vi "Reserve Registered Sessions.vi"(6 "timeout (ms)":i32, 8 "error in (no error)":errorcluster, 9 "instrument type id":string) -> (0 "error out":errorcluster, 3 "session reservation out":refnum<class "Session Reservation.lvclass">)   [LabVIEW 2020, in "MeasurementLink Session Management.lvlib" / "Session Reservation.lvclass"]
doc: "Reserves all registered session(s) with the specified <b>instrument type id</b>. If the <b>instrument type id</b> is an empty string, reserves all registered sessions for all instrument types."
uses:
  Session Reservation.lvclass
  MeasurementLink Session Management Client/RPC Messages/ni_measurementlink_sessionmanagement_v1_ReserveAllRegisteredSessionsRequest.ctl
  MeasurementLink Session Management Client/RPC Messages/ni_measurementlink_PinMapContext.ctl
  IReservationObserver/IReservationObserver.lvclass
  Session Reservation.lvclass/Session Reservation.ctl
  MeasurementLink Session Management Client/MeasurementLink Session Management Client.lvlib
  MeasurementLink Session Management Client Wrapper/MeasurementLink Session Management Client Wrapper.lvlib
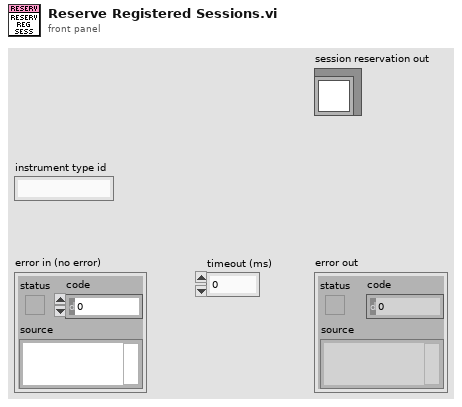
[diagram p1: front panel]
types:
  T1 = typedef "MeasurementLink Session Management Client.lvlib/ni_measurementlink_PinMapContext.ctl" = cluster{"pin_map_id":string, "sites":i32[]}
  T2 = typedef "MeasurementLink Session Management Client.lvlib/ni_measurementlink_sessionmanagement_v1_ReserveAllRegisteredSessionsRequest.ctl" = cluster{"timeout_in_milliseconds":i32, "instrument_type_id":string}
  T3 = typedef "MeasurementLink Session Management Client.lvlib/ni_measurementlink_sessionmanagement_v1_ReserveAllRegisteredSessionsResponse.ctl" = cluster{"sessions":T4[]}
  T4 = typedef "MeasurementLink Session Management Client.lvlib/ni_measurementlink_sessionmanagement_v1_SessionInformation.ctl" = cluster{"session":T5, "resource_name":string, "channel_list":string, "instrument_type_id":string, "session_exists":bool, "channel_mappings":T6[]}
  T5 = typedef "MeasurementLink Session Management Client.lvlib/nidevice_grpc_Session.ctl" = cluster{"name":string}
  T6 = typedef "MeasurementLink Session Management Client.lvlib/ni_measurementlink_sessionmanagement_v1_ChannelMapping.ctl" = cluster{"pin_or_relay_name":string, "site":i32, "channel":string}
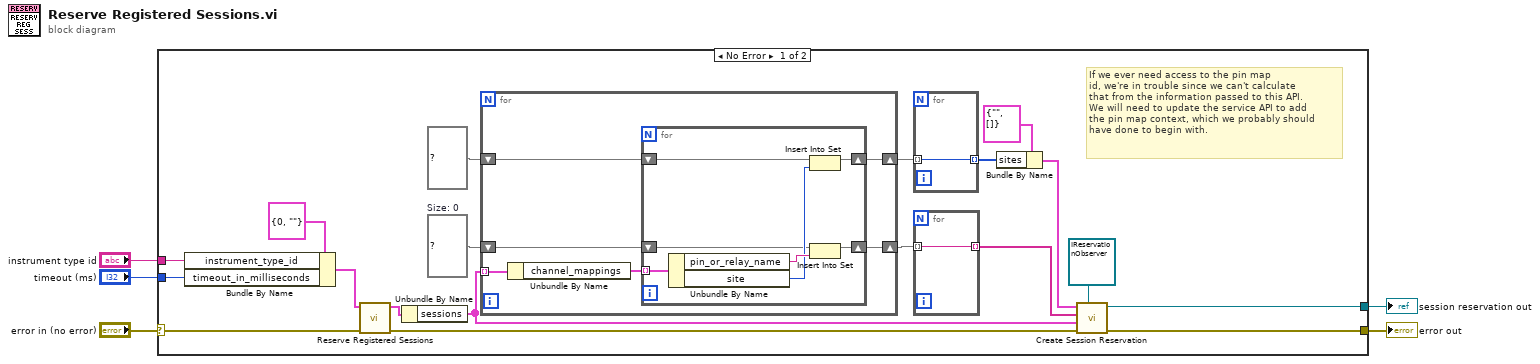
[diagram p0: block diagram]
diagram:
  n1 = case shown="No Error" "error in (no error)" {
    selector: "error in (no error)" -> [w23 w40]
    tunnel: "instrument type id" -> [w22 _]
    tunnel: "timeout (ms)" -> [w21 _]
    tunnel: [w19 _] -> w3
    tunnel: [w17 w40] -> w4
    frame No Error {
      w13 = set{string} {}  # Size: 0
      # "If we ever need access to the pin map\nid, we're in trouble since we can't calculate\nthat from the information passed to this API.\nWe will need to update the service API to add\nthe pin map context, which we probably should\nhave done to begin with."
      n2 = Bundle By Name(cluster=T2 {"timeout_in_milliseconds"=0, "instrument_type_id"=""} ("Request Data"), "instrument_type_id"=w22, "timeout_in_milliseconds"=w21) -> (w20:T2)
      n3 = call "Reserve Registered Sessions.vi"("error in"=w23, "request data"=w20) -> ("error out"=w18:errorcluster, "response data"=w16:T3)  [unwired: 8 in]
      n4 = Unbundle By Name(w16) -> ("sessions"=w15:T4[])
      n5 = for {
        tunnel: w15 -> [w32] mode=indexing
        shift-right: [w28] -> w12
        shift-left: w13 -> [w27]
        shift-right: [w29] -> w11
        shift-left: set{i32} {} ("set in") -> [w30]
        n6 = Unbundle By Name(w32) -> ("channel_mappings"=w31:T6[])
        n7 = for {
          tunnel: w31 -> [w39] mode=indexing
          shift-right: [w34] -> w28
          shift-left: w27 -> [w33]
          shift-right: [w35] -> w29
          shift-left: w30 -> [w36]
          n8 = Unbundle By Name(w39) -> ("pin_or_relay_name"=w38:string, "site"=w37:i32)
          n9 = Insert Into Set(10:w37, 11:w36) -> (3:w35:set{i32})  [unwired: 1 out]
          n10 = Insert Into Set(10:w38, 11:w33) -> (3:w34:set{string})  [unwired: 1 out]
        }
      }
      n11 = for {
        tunnel: [w25] -> w8 mode=indexing
        tunnel: w11 -> [w25] mode=indexing
      }
      n12 = for {
        tunnel: [w26] -> w10 mode=indexing
        tunnel: w12 -> [w26] mode=indexing
      }
      n13 = Bundle By Name(cluster=T1 {"pin_map_id"="", "sites"=[]} ("pin map context"), "sites"=w8) -> (w7:T1)
      n14 = call "Create Session Reservation.vi"("reservation observer"=refnum<class "IReservationObserver.lvclass"> refnum, "error in (no error)"=w18, "sessions"=w15, "pin or relay names"=w10, "pin map context"=w7) -> ("error out"=w17:errorcluster, "session reservation out"=w19:refnum<class "Session Reservation.lvclass">)  [unwired: 5 in]
    }
    frame Error {
    }
  }
  "error out" <- w4
  "session reservation out" <- w3
